vi "Counter(NI-6009).vi"() -> ()   [LabVIEW 2015]
uses:
  <vilib>/Utility/error.llb/DialogType.ctl
  <vilib>/DAQmx/read.llb/DAQmx Read (Counter U32 1Chan 1Samp).vi
  <vilib>/DAQmx/create/channels.llb/DAQmx Create Channel (CI-Count Edges).vi
  <vilib>/DAQmx/miscellaneous.llb/DAQmx Fill In Error Info.vi
  <resource>/objmgr/daqmx.rc
panel:
  in  "counter":tag="Dev2/ctr0"
  in  "y":bool
  in  "CI.CountEdges.Term":tag
  in  "CI.CountEdges.ActiveEdge":i32(ring)=10280 items=["Rising"=10280, "Falling"=10171]
  in  "milliseconds to wait":u32
  out "data":u32
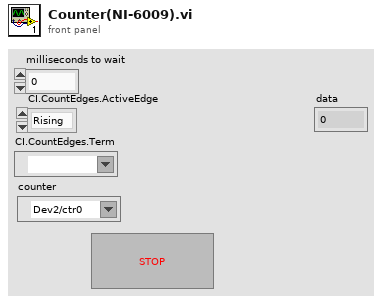
[diagram p1: front panel]
types:
  T1 = typedef "DialogType.ctl" = u16
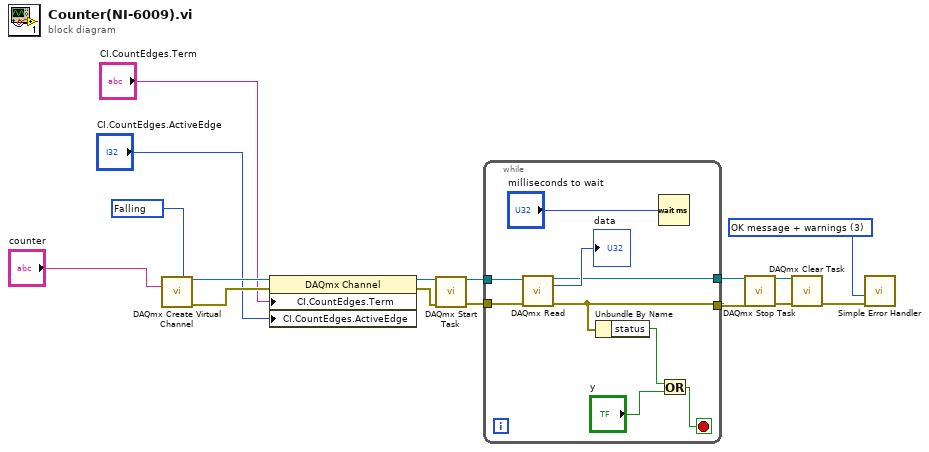
[diagram p0: block diagram]
diagram:
  w1 = 10171 items=["Rising"=10280, "Falling"=10171] ("edge")
  w4 = T1 3 items=["no dialog", "OK message", "continue or stop message", "OK message + warnings", "continue/stop + warnings"] ("type of dialog (OK msg:1)")
  n1 = call-poly <vilib>:"DAQmx Create Virtual Channel.vi"("edge"=w1, "counter"="counter") -> ("task out"=w15:refnum<k21>, "error out"=w14:errorcluster)  [unwired: 12 in]
  n2 = property class="DAQmx Channel"(reference=w15, error in=w14, "CI.CountEdges.Term"="CI.CountEdges.Term", "CI.CountEdges.ActiveEdge"="CI.CountEdges.ActiveEdge") -> (reference out=w13:refnum<k21>, error out=w12:errorcluster)
  n3 = call <vilib>:"DAQmx Start Task.vi"("task/channels in"=w13, "error in"=w12) -> ("task out"=w11:refnum<k21>, "error out"=w10:errorcluster)  [unwired: 12 in]
  n4 = while {
    tunnel: w11 -> [w25]
    tunnel: w10 -> [w24]
    tunnel: [w22] -> w8
    tunnel: [w21] -> w9
    stop <- w19 stop-if-true
    n5 = call-poly <vilib>:"DAQmx Read.vi"("task/channels in"=w25, "error in"=w24) -> ("task out"=w21:refnum<k21>, "data"=→"data":u32, "error out"=w22:errorcluster)  [unwired: 11 in]
    n6 = Unbundle By Name(w22) -> ("status"=w18:bool)
    n7 = Wait (ms)(milliseconds to wait="milliseconds to wait") -> ()  [unwired: 1 out]
    n8 = Or(x=w18, y="y") -> (x .or. y?=w19:bool)
  }
  n9 = call <vilib>:"DAQmx Stop Task.vi"("task/channels in"=w9, "error in"=w8) -> ("task out"=w7:refnum<k21>, "error out"=w6:errorcluster)  [unwired: 12 in]
  n10 = call <vilib>:"DAQmx Clear Task.vi"("task in"=w7, "error in"=w6) -> ("error out"=w5:errorcluster)  [unwired: 13 in]
  n11 = call <vilib>:"Simple Error Handler.vi"("type of dialog (OK msg:1)"=w4, "error in (no error)"=w5) -> ()  [unwired: 3 in, 5 out]
